vi "read_temps.vi"() -> ()   [LabVIEW 2015]
uses:
  <vilib>/Analysis/baseanly.llb/Mean (DBL).vi
  <vilib>/Analysis/NI_AALBase.lvlib
panel:
  in  "index (row)":i32
  out "Tplate":dbl format="%0.4f"
  # "Runs until all_stop is asserted\nTemperature is published on shared variable \nTplate"
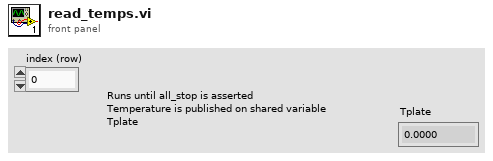
[diagram p1: front panel]
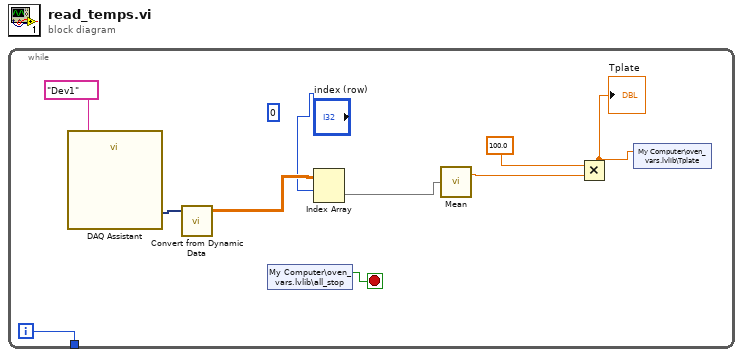
[diagram p0: block diagram]
diagram:
  n1 = while {
    tunnel: [w1] -> _
    i -> [w1]
    stop <- w3 stop-if-true
    (unwired) 0 ("index")
    n2 = call "DAQ Assistant"("device name"=tag "Dev1") -> ("data"=w7:dynamicdata)  [unwired: 15 in, 3 out]
    n3 = call "Convert from Dynamic Data"("Dynamic Data Type"=w7) -> ("Array"=w5:dbl[][])  [unwired: 3 in]
    n4 = shared-variable "My Computer\\oven_vars.lvlib\\all_stop"() -> (w3:bool)  [unwired: 1 in, 1 out]
    n5 = Index Array(array=w5, index (row)="index (row)") -> (element=w10:dbl[])  [unwired: 1 in]
    n6 = call-poly <vilib>:"Mean.vi"("X"=w10) -> ("mean"=w9:dbl)  [unwired: 1 out]
    n7 = Multiply(x=100.0, y=w9) -> (x*y=w4:dbl)
    "Tplate" <- w4
    n8 = shared-variable "My Computer\\oven_vars.lvlib\\Tplate"(w4) -> ()  [unwired: 1 in, 1 out]
  }
